vi "OW Write Read Bytes.vi"(4 "IntervalTimeUs":u32, 5 "ReadDataLen":u32, 6 "pReadData":u8[](array[numeric])=array[4097 elements], 7 "WriteDataLen":u32, 9 "pWriteData":u8, 10 "ChannelMask":u32, 11 "DevHandle":i32) -> (1 "pWriteData out":u8, 2 "function return":i32, 3 "pReadData out":u8[](array[numeric]))   [LabVIEW 2010, in "usb2ow.lvlib"]
doc: "int WINAPI OW_WriteReadBytes(int DevHandle, unsigned int ChannelMask,unsigned char *pWriteData,unsigned int WriteDataLen,unsigned char *pReadData,unsigned int ReadDataLen,unsigned int IntervalTimeUs);"
uses:
  usb2ow.lvlib
  USB2XXX/trunk/USB2XXX/USB2XXX/vs2010/Release/USB2XXX.dll
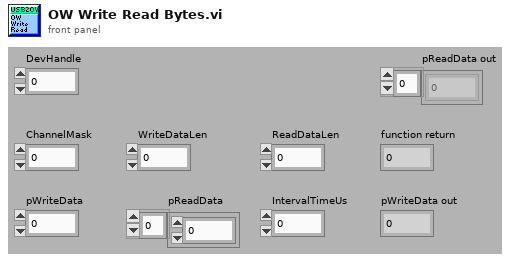
[diagram p1: front panel]
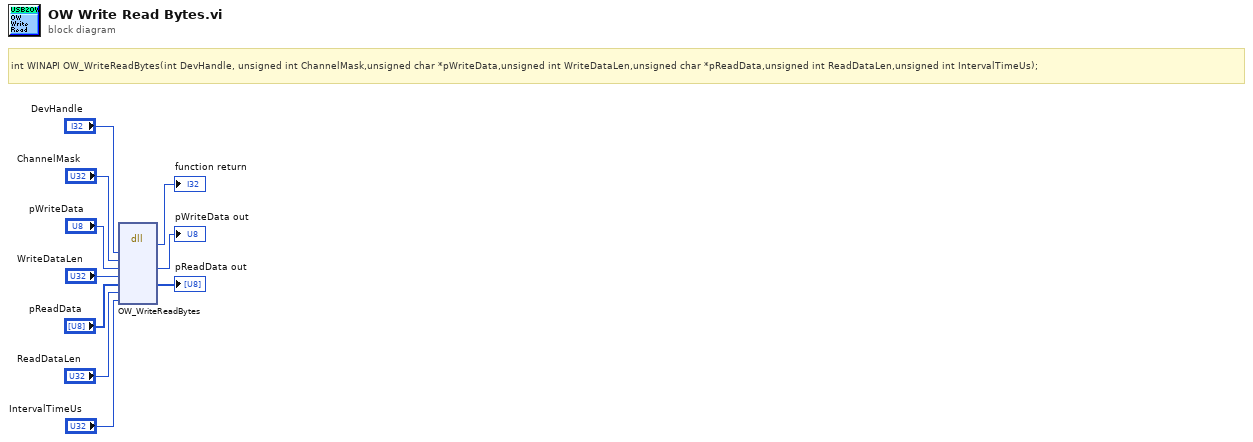
[diagram p0: block diagram]
diagram:
  # "int WINAPI OW_WriteReadBytes(int DevHandle, unsigned int ChannelMask,unsigned char *pWriteData,unsigned int WriteDataLen,unsigned char *pReadData,unsigned int ReadDataLen,unsigned int IntervalTimeUs);"
  n1 = dll-call lib="E:/OtherWork/STM32/USB2XXX/trunk/USB2XXX/USB2XXX/vs2010/Release/USB2XXX.*" fn="OW_WriteReadBytes"("DevHandle"="DevHandle", "ChannelMask"="ChannelMask", "pWriteData"="pWriteData", "WriteDataLen"="WriteDataLen", "pReadData"="pReadData", "ReadDataLen"="ReadDataLen", "IntervalTimeUs"="IntervalTimeUs") -> (→"function return":i32, "pWriteData"=→"pWriteData out":u8, "pReadData"=→"pReadData out":u8[])  [unwired: 8 in, 2 out]
